vi "CardMuxSwitch.vi"(6 "disabled channels":u32[](array[numeric]), 8 "error in (no error)":errorcluster, 10 "Switch to channel":i32) -> (0 "error out":errorcluster)   [LabVIEW 2013]
uses:
  general_VIs/globals/QC_MeasurementSetup.vi
  InstrControl/InstrumentSetup.vi
  InstrControl/InstrControl.lvclass
  InstrControl/Switching/Switching.lvclass
panel:
  out "last channel no.":i32
  out "Display Matrix":bool[][](array[boolean])
  # "Pickering Multiplexer Settings"
  # "X1"
  # "X2"
  # "X3"
  # "X4"
  # "X5"
  # "X6"
  # "X7"
  # "X8"
  # "Y1  Y2  Y3  Y4"
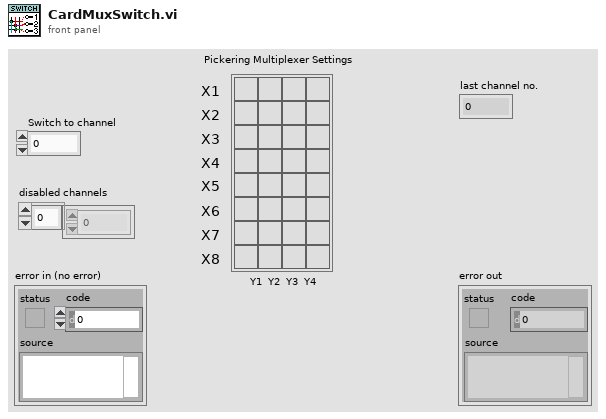
[diagram p1: front panel]
types:
  T1 = cluster{"Bias Supply":refnum<class "SupplyControl.lvclass">, "SMU":refnum<class "SupplyControl.lvclass">, "LCR":refnum<class "LCRControl.lvclass">, "Probe Card Channels":i32, "Bias Voltage [V]":dbl, "First strip":i32, "Last strip":i32, "Base Voltage [V]":dbl, "Base Ramp Step [V]":dbl, "Base Ramp Interval [s]":dbl, "High Voltage [V]":dbl, "High Ramp Step [V]":dbl, "High Ramp Interval [s]":dbl, "Single Needle":bool, "ArduinoControl.lvclass":refnum<class "ArduinoControl.lvclass">, "Fraction of good strips [%]":dbl}
  T2 = cluster{"GPIB address":string, "Matrix address":string, "Mux1 address":string, "Mux2 address":string, "Matrix used?":bool, "Switching":refnum<class "Switching.lvclass">, "Matrix X Channels":cluster{"Bias Supply / SMU LO":i32, "Bias Supply / SMU HI":i32, "CV Box LO":i32, "CV Box HI":i32, "CV Box LO IN":i32, "CV Box HI IN":i32, "Volt meter LO":i32, "Volt meter HI":i32, "Mux1 C1":i32, "Mux1 C2":i32, "Mux2 C1":i32, "Mux2 C2":i32}}
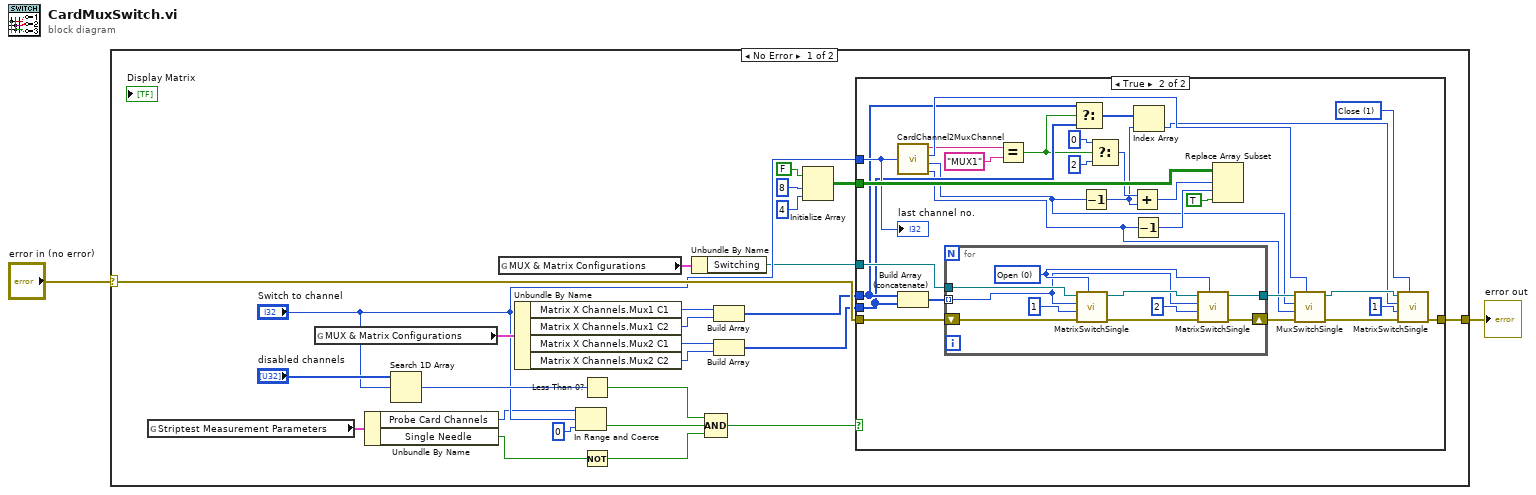
[diagram p0: block diagram]
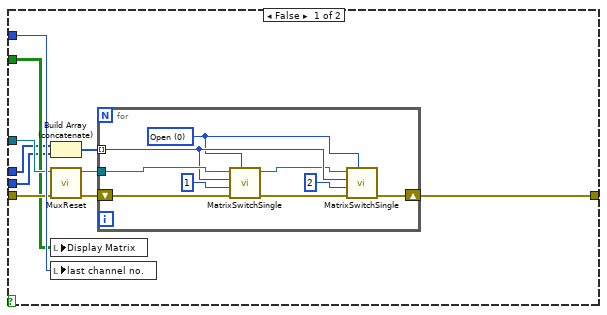
[diagram p2: hidden frame]
diagram:
  n1 = case shown="No Error" "error in (no error)" {
    selector: "error in (no error)" -> [w26 w87]
    tunnel: [w21 w87] -> w1
    frame No Error {
      n2 = global read "QC_MeasurementSetup.vi" "Striptest Measurement Parameters"() -> (w28:T1)
      n3 = global read "InstrumentSetup.vi" "MUX & Matrix Configurations"() -> (w27:T2)
      n4 = Unbundle By Name(w28) -> ("Probe Card Channels"=w5:i32, "Single Needle"=w15:bool)
      n5 = Search 1D Array(1D array="disabled channels", element="Switch to channel") -> (index of element=w18:i32)  [unwired: 1 in]
      n6 = global read "InstrumentSetup.vi" "MUX & Matrix Configurations"() -> (w4:T2)
      n7 = Unbundle By Name(w27) -> ("Matrix X Channels.Mux1 C1"=w23:i32, "Matrix X Channels.Mux1 C2"=w22:i32, "Matrix X Channels.Mux2 C1"=w24:i32, "Matrix X Channels.Mux2 C2"=w25:i32)
      n8 = In Range and Coerce(upper limit=w5, x="Switch to channel", lower limit=0) -> (In Range?=w16:bool)  [unwired: 1 out]
      n9 = Less Than 0?(x=w18) -> (x < 0?=w17:bool)
      n10 = Not(x=w15) -> (.not. x?=w14:bool)
      n11 = Unbundle By Name(w4) -> ("Switching"=w3:refnum<class "Switching.lvclass">)
      n12 = Compound Arithmetic op=AND(w17, w16, w14) -> (w13:bool)
      n13 = Build Array(w23, w22) -> (w7:i32[])
      n14 = Build Array(w24, w25) -> (w6:i32[])
      n15 = Initialize Array(FALSE, 8, 4) -> (w8:bool[][])
      n16 = case shown="True" w13 {
        tunnel: "Switch to channel" -> [w38 w67]
        tunnel: w3 -> [w37 w76]
        tunnel: w26 -> [w34 w75]
        tunnel: [w33 w56] -> w21
        tunnel: w8 -> [w32 w68]
        tunnel: w7 -> [w31 w61]
        tunnel: w6 -> [w30 w60]
        frame False {
          n17 = Build Array (concatenate)(w31, w30) -> (w29:i32[])
          n18 = call "MuxReset.vi"("error in (no error)"=w34, "Switching in"=w37) -> ("error out"=w35:errorcluster, "Switching out"=w36:refnum<class "Switching.lvclass">)  [unwired: 8 in]
          n19 = local write "Display Matrix"(w32) -> ()
          n20 = local write "last channel no."(w38) -> ()
          n21 = for {
            tunnel: w36 -> [w47]
            tunnel: w29 -> [w45] mode=indexing
            shift-right: [w44] -> w33
            shift-left: w35 -> [w46]
            w43 = u16 0 items=["Open", "Close"] ("Switch action")
            n22 = call "MatrixSwitchSingle.vi"("Switch action"=w43, "error in (no error)"=w46, "Matrix Y"=1, "Matrix X"=w45, "Switching in"=w47) -> ("error out"=w41:errorcluster, "Switching out"=w42:refnum<class "Switching.lvclass">)  [unwired: 4 in, 1 out]
            n23 = call "MatrixSwitchSingle.vi"("Switch action"=w43, "error in (no error)"=w41, "Matrix Y"=2, "Matrix X"=w45, "Switching in"=w42) -> ("error out"=w44:errorcluster)  [unwired: 4 in, 2 out]
          }
        }
        frame True {
          w72 = u16 1 items=["Open", "Close"] ("Switch action")
          n24 = call "CardChannel2MuxChannel.vi"("Probecard Channel No."=w67) -> ("Mux No. string"=w62:string, "Mux No.:"=w64:u32, "C1 / C2"=w50:i32, "Channel"=w55:i32)
          n25 = Build Array (concatenate)(w61, w60) -> (w59:i32[])
          n26 = for {
            tunnel: w76 -> [w83]
            tunnel: w59 -> [w80] mode=indexing
            shift-right: [w84] -> w66
            shift-left: w75 -> [w86]
            tunnel: [w77] -> w65
            w81 = u16 0 items=["Open", "Close"] ("Switch action")
            n27 = call "MatrixSwitchSingle.vi"("Switch action"=w81, "error in (no error)"=w86, "Matrix Y"=1, "Matrix X"=w80, "Switching in"=w83) -> ("error out"=w85:errorcluster, "Switching out"=w82:refnum<class "Switching.lvclass">)  [unwired: 4 in, 1 out]
            n28 = call "MatrixSwitchSingle.vi"("Switch action"=w81, "error in (no error)"=w85, "Matrix Y"=2, "Matrix X"=w80, "Switching in"=w82) -> ("error out"=w84:errorcluster, "Switching out"=w77:refnum<class "Switching.lvclass">)  [unwired: 4 in, 1 out]
          }
          n29 = Equal?(x=w62, y="MUX1") -> (x = y?=w54:bool)
          n30 = Select(t=w61, s=w54, f=w60) -> (s? t:f=w58:i32[])
          n31 = Decrement(x=w50) -> (x-1=w48:i32)
          n32 = Select(t=0, s=w54, f=2) -> (s? t:f=w51:i32)
          n33 = Add(x=w51, y=w48) -> (x+y=w49:i32)
          n34 = Decrement(x=w55) -> (x-1=w70:i32)
          n35 = Index Array(array=w58, index=w48) -> (element=w57:i32)
          n36 = Replace Array Subset(array=w68, new element=TRUE, index (row)=w49, index (col)=w70) -> ()  [unwired: 1 out]
          n37 = call "MuxSwitchSingle.vi"("MUX address"=w64, "error in (no error)"=w66, "Channel"=w55, "C1 / C2"=w50, "Switching in"=w65) -> ("error out"=w74:errorcluster, "Switching out"=w73:refnum<class "Switching.lvclass">)  [unwired: 4 in, 1 out]
          n38 = call "MatrixSwitchSingle.vi"("Switch action"=w72, "error in (no error)"=w74, "Matrix Y"=1, "Matrix X"=w57, "Switching in"=w73) -> ("error out"=w56:errorcluster)  [unwired: 4 in, 2 out]
          "last channel no." <- w67
        }
      }
    }
    frame Error {
    }
  }
  "error out" <- w1
